vi "get_covariance.vi"(8 "error in (no error)":errorcluster, 11 "Interface_get_covariance in":refnum<class "Interface_get_covariance.lvclass">) -> (0 "error out":errorcluster, 2 "cov":dbl[][](array[numeric]), 3 "Interface_get_covariance out":refnum<class "Interface_get_covariance.lvclass">)   [LabVIEW 2020, in "Interface_get_covariance.lvclass"]
doc: "Return the covariance."
uses:
  Interface_get_covariance.lvclass
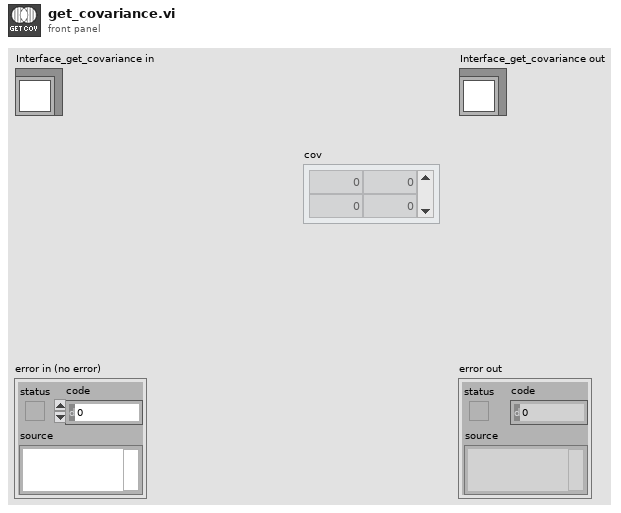
[diagram p1: front panel]
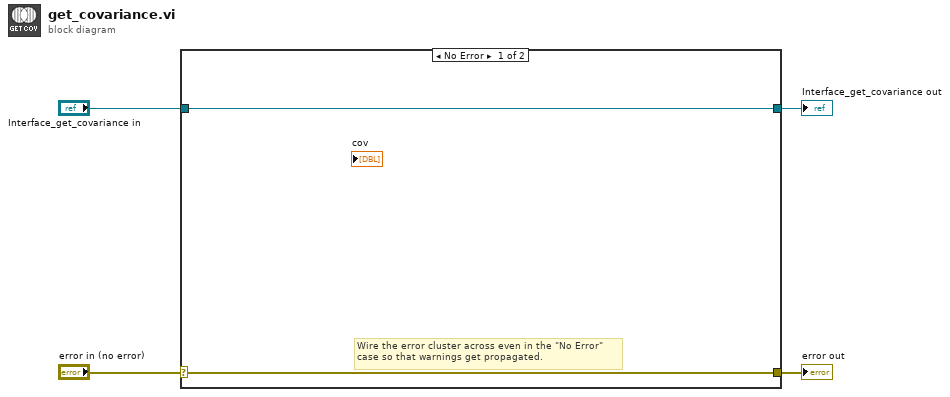
[diagram p0: block diagram]
diagram:
  n1 = case shown="No Error" "error in (no error)" {
    selector: "error in (no error)" -> [w5 w8]
    tunnel: [w5 w8] -> w3
    tunnel: [w6 w7] -> w1
    tunnel: "Interface_get_covariance in" -> [w6 w7]
    frame No Error {
      # "Wire the error cluster across even in the \"No Error\"\ncase so that warnings get propagated."
    }
    frame Error {
    }
  }
  "error out" <- w3
  "Interface_get_covariance out" <- w1
